vi "Write Material Movement CEID.vi"(8 "error in (no error)":errorcluster, 10 "Material Movement CEID":u32, 11 "21-Material Movement in":refnum<class "21-Material Movement.lvclass">) -> (0 "error out":errorcluster, 3 "21-Material Movement out":refnum<class "21-Material Movement.lvclass">)   [LabVIEW 2020, in "SECS Scenarios.lvlib" / "21-Material Movement.lvclass"]
uses:
  21-Material Movement.lvclass
  21-Material Movement.lvclass/21-Material Movement.ctl
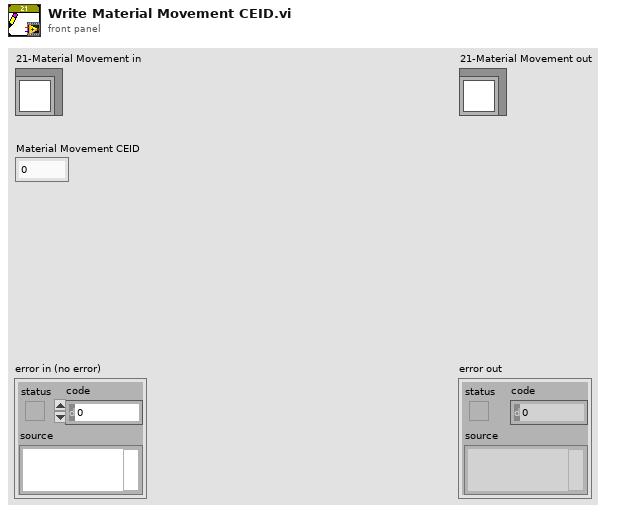
[diagram p1: front panel]
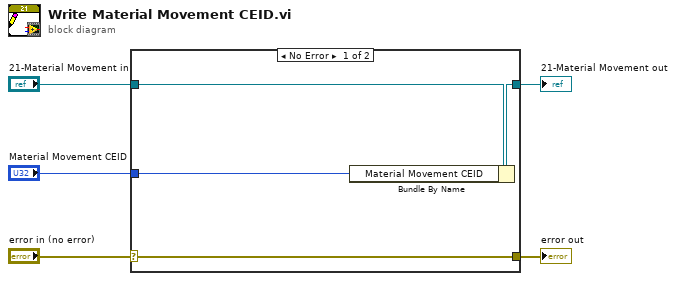
[diagram p0: block diagram]
diagram:
  n1 = case shown="No Error" "error in (no error)" {
    selector: "error in (no error)" -> [w9 w10]
    tunnel: [w9 w10] -> w4
    tunnel: [w7 w11] -> w2
    tunnel: "21-Material Movement in" -> [w8 w11]
    tunnel: "Material Movement CEID" -> [w6 _]
    frame No Error {
      n2 = Bundle By Name(cluster=w8, "Material Movement CEID"=w6) -> (w7:refnum<class "21-Material Movement.lvclass">)
    }
    frame Error {
    }
  }
  "error out" <- w4
  "21-Material Movement out" <- w2
